vi "PI_valvulas5.vi"(8 "Temperatura manifold":dbl format="%.2f", 9 "controlON":bool, 10 "Temperatura bobina":dbl format="%.2f", 11 "Setpoint T":dbl) -> (3 "PWM (%)":dbl)   [LabVIEW 2022 SP3, in "DAQ_Termopares.lvlib"]
uses:
  DAQ/DAQ_Termopares.lvlib
  <vilib>/addons/control/pid/pid.llb/PID (DBL).vi
  <vilib>/addons/control/pid/NI_PID_pid.lvlib
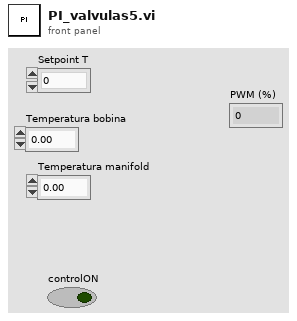
[diagram p1: front panel]
types:
  T1 = cluster{"proportional gain (Kc)":dbl, "integral time (Ti, min)":dbl, "derivative time (Td, min)":dbl}
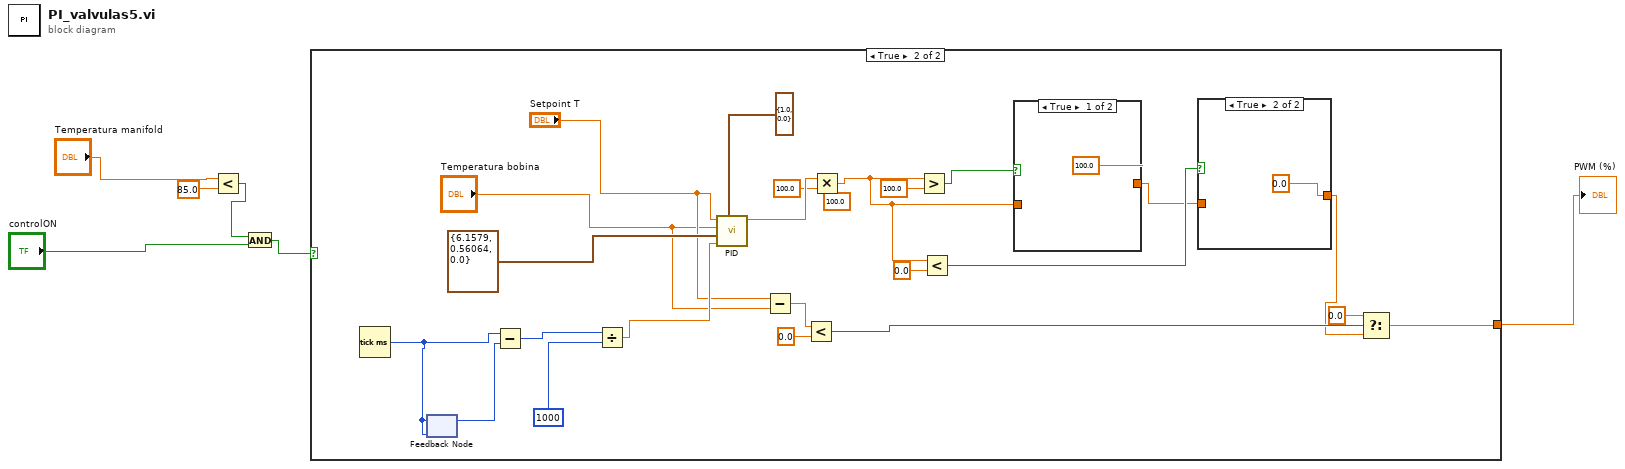
[diagram p0: block diagram]
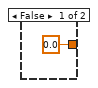
[diagram p2: hidden frame]
diagram:
  n1 = Less?(x="Temperatura manifold", y=85.0) -> (x < y?=w2:bool)
  n2 = And(x=w2, y="controlON") -> (x .and. y?=w6:bool)
  n3 = case shown="True" w6 {
    tunnel: [0.0 ("t") w8] -> w1
    frame False {
    }
    frame True {
      (unwired) 100.0 ("y")
      n4 = Tick Count (ms)() -> (millisecond timer value=w30:u32)
      n5 = feedback #1(w30) -> (w29:u32)
      n6 = feedback-in #1(w30) -> ()
      n7 = Subtract(x=w30, y=w29) -> (x-y=w27:u32)
      n8 = Divide(x=w27, y=1000) -> (x/y=w16:dbl)
      n9 = call-poly <vilib>:"PID.vi"("output range"=cluster{"output high":dbl, "output low":dbl} {"output high"=1.0, "output low"=0.0}, "dt (s)"=w16, "PID gains"=T1 {"proportional gain (Kc)"=6.1579, "integral time (Ti, min)"=0.56064, "derivative time (Td, min)"=0.0}, "process variable"="Temperatura bobina", "setpoint"="Setpoint T") -> ("output"=w24:dbl)  [unwired: 5 in, 1 out]
      n10 = Subtract(x="Setpoint T", y="Temperatura bobina") -> (x-y=w13:dbl)
      n11 = Less?(x=w13, y=0.0) -> (x < y?=w11:bool)
      n12 = Multiply(x=w24, y=100.0) -> (x*y=w19:dbl)
      n13 = Greater?(x=w19, y=100.0) -> (0:w20:bool)
      n14 = Less?(x=w19, y=0.0) -> (x < y?=w18:bool)
      n15 = case shown="True" w20 {
        tunnel: w19 -> [_ w34]
        tunnel: [100.0 w34] -> w17
        frame True {
        }
        frame False {
        }
      }
      n16 = case shown="True" w18 {
        tunnel: w17 -> [w31 _]
        tunnel: [w31 0.0] -> w9
        frame False {
        }
        frame True {
        }
      }
      n17 = Select(t=0.0, s=w11, f=w9) -> (s? t:f=w8:dbl)
    }
  }
  "PWM (%)" <- w1
